vi "add_range.vi"(5 "Range Data":T1, 6 "Stamp":cluster{"frame_id":string, "reset seq?":bool}, 7 "msg in":string) -> (3 "msg out":string)   [LabVIEW 2015]
uses:
  std_msgs/subs/u8Scalar.vi
  std_msgs/subs/float32Scalar.vi
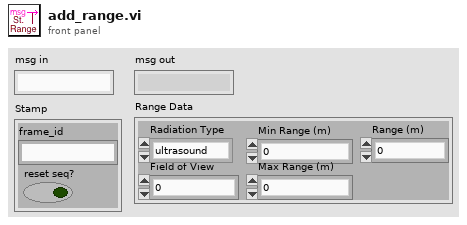
[diagram p1: front panel]
types:
  T1 = cluster{"Radiation Type":enum16{"ultrasound", "infrared"}, "Field of View":sgl, "Min Range (m)":sgl, "Max Range (m)":sgl, "Range (m)":sgl}
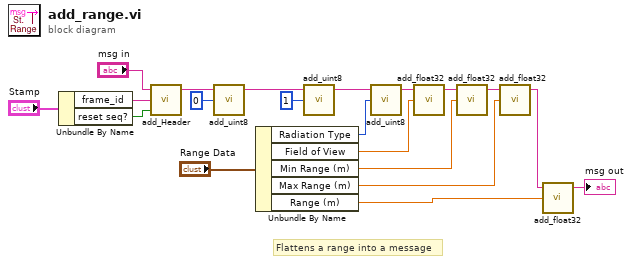
[diagram p0: block diagram]
diagram:
  # "Flattens a range into a message"
  n1 = Unbundle By Name("Stamp") -> ("frame_id"=w8:string, "reset seq?"=w7:bool)
  n2 = call "add_Header.vi"("reset seq?"=w7, "frame_id"=w8, "msg in"="msg in") -> ("msg out"=w18:string)  [unwired: 2 in]
  n3 = call-poly "add_uint8.vi"("Numeric"=u8 0, "msg in"=w18) -> ("msg out"=w17:string)  [unwired: 3 in]
  n4 = Unbundle By Name("Range Data") -> ("Radiation Type"=w5:enum16{"ultrasound", "infrared"}, "Field of View"=w4:sgl, "Min Range (m)"=w3:sgl, "Max Range (m)"=w2:sgl, "Range (m)"=w1:sgl)
  n5 = call-poly "add_uint8.vi"("Numeric"=u8 1, "msg in"=w17) -> ("msg out"=w16:string)  [unwired: 3 in]
  n6 = call-poly "add_uint8.vi"("Numeric"=w5, "msg in"=w16) -> ("msg out"=w15:string)  [unwired: 3 in]
  n7 = call-poly "add_float32.vi"("Numeric"=w4, "msg in"=w15) -> ("msg out"=w14:string)  [unwired: 3 in]
  n8 = call-poly "add_float32.vi"("Numeric"=w3, "msg in"=w14) -> ("msg out"=w19:string)  [unwired: 3 in]
  n9 = call-poly "add_float32.vi"("Numeric"=w2, "msg in"=w19) -> ("msg out"=w13:string)  [unwired: 3 in]
  n10 = call-poly "add_float32.vi"("Numeric"=w1, "msg in"=w13) -> ("msg out"=→"msg out":string)  [unwired: 3 in]
